vi "REV Sequence.vi"() -> ()   [LabVIEW 2026]
uses:
  <vilib>/REVLibDriver5/subvi/RevLibError.ctl
  <vilib>/Custom Controls/c_Spark_MotorType.ctl
  <vilib>/REVLibDriver5/REVLibDriver.lvlib
  <vilib>/Custom Controls/c_Spark_SparkModel.ctl
  lib/libREVLibDriver.so
panel:
  out "c_Spark_SparkModel":T1 items=["c_Spark_Unknown", "c_Spark_SparkFlex", "c_Spark_SparkMax"]
  out "function return 4":T2
  out "fwVersion out":T3
  in  "stop":bool
  out "function return 3":T2
  out "function return 2":T2
  out "function return":T2
  out "deviceId out":i32
  out "status out":T2
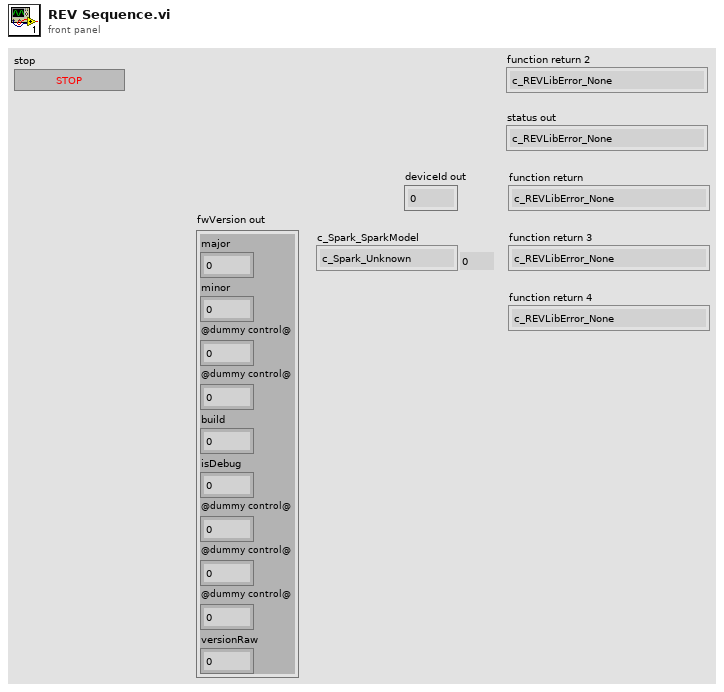
[diagram p1: front panel]
types:
  T1 = typedef "REVLibDriver.lvlib/c_Spark_SparkModel.ctl" = u16
  T2 = typedef "REVLibDriver.lvlib/RevLibError.ctl" = enum16{"c_REVLibError_None", "c_REVLibError_General", "c_REVLibError_CANTimeout", "c_REVLibError_NotImplemented", "c_REVLibError_HAL", "c_REVLibError_CantFindFirmware", "c_REVLibError_FirmwareTooOld", "c_REVLibError_FirmwareTooNew", "c_REVLibError_ParamInvalidID", "c_REVLibError_ParamMismatchType", "c_REVLibError_ParamAccessMode", "c_REVLibError_ParamInvalid", "c_REVLibError_ParamNotImplementedDeprecated", "c_REVLibError_FollowConfigMismatch", "c_REVLibError_Invalid", "c_REVLibError_SetpointOutOfRange", "c_REVLibError_Unknown", "c_REVLibError_CANDisconnected", "c_REVLibError_DuplicateCANId", "c_REVLibError_InvalidCANId", "c_REVLibError_SparkMaxDataPortAlreadyConfiguredDifferently", "c_REVLibError_SparkFlexBrushedWithoutDock", "c_REVLibError_InvalidBrushlessEncoderConfiguration", "c_REVLibError_FeedbackSensorIncompatibleWithDataPortConfig", "c_REVLibError_ParamInvalidChannel", "c_REVLibError_ParamInvalidValue", "c_REVLibError_CannotPersistParametersWhileEnabled", "c_REVLibError_NotReadyToReceiveCommand", "c_REVLibError_NumCodes"}
  T3 = cluster{"major":u8, "minor":u8, "@dummy control@":i8, "@dummy control@":i8, "build":u32, "isDebug":u8, "@dummy control@":i8, "@dummy control@":i8, "@dummy control@":i8, "versionRaw":u32}
  T4 = typedef "REVLibDriver.lvlib/c_Spark_MotorType.ctl" = enum16{"c_Spark_kMotorType_BRUSHED", "    c_Spark_kMotorType_BRUSHLESS", "    c_Spark_kNumMotorTypes"}
  T5 = typedef "REVLibDriver.lvlib/c_Spark_handle.ctl" = cluster{"Pointer":u64}
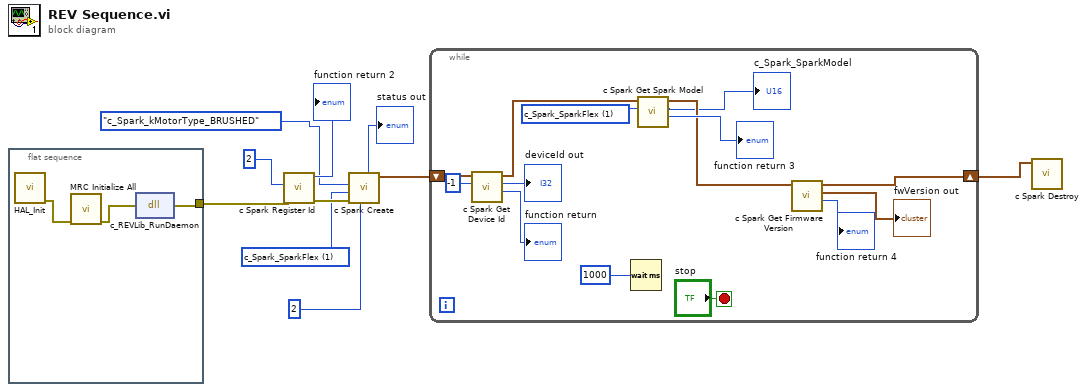
[diagram p0: block diagram]
diagram:
  w9 = T1 1 items=["c_Spark_SparkMax"=0, "c_Spark_SparkFlex"=1, "c_Spark_Unknown"=255] ("unconfirmedModel")
  n1 = flat-sequence {
    tunnel: [w13] -> w3
    frame #0 {
      n2 = call "HAL_Init.vi"() -> ("error out"=w12:errorcluster)  [unwired: 11 in]
      n3 = call <vilib>:"MRC Initialize All.vi"("error out 2"=w12) -> ("error out"=w11:errorcluster)  [unwired: 10 in]
      n4 = dll-call lib="home/systemcore/natinst/lib/libREVLibDriver.so" fn="c_REVLib_RunDaemon"(error in=w11) -> (error out=w13:errorcluster)  [unwired: 3 in, 1 out]
    }
  }
  n5 = call <vilib>:"c Spark Register Id.vi"("error in (no error)"=w3, "deviceId"=2) -> ("error out"=w10:errorcluster, "function return"=→"function return 2":T2)  [unwired: 8 in]
  n6 = call <vilib>:"c Spark Create.vi"("deviceId"=2, "error in (no error)"=w10, "unconfirmedModel"=w9, "type"=c_Spark_MotorType."c_Spark_kMotorType_BRUSHED") -> ("handle"=w6:T5, "status out"=→"status out":T2)  [unwired: 5 in, 1 out]
  n7 = while {
    shift-right: [w15] -> w2
    shift-left: w6 -> [w27]
    stop <- "stop" stop-if-true
    w16 = T1 1 items=["c_Spark_Unknown", "c_Spark_SparkFlex", "c_Spark_SparkMax"] ("model")
    n8 = call <vilib>:"c Spark Get Device Id.vi"("deviceId"=-1, "handle"=w27) -> ("function return"=→"function return":T2, "deviceId out"=→"deviceId out":i32, "handle out"=w24:T5)  [unwired: 6 in, 1 out]
    n9 = Wait (ms)(milliseconds to wait=u32 1000) -> ()  [unwired: 1 out]
    n10 = call <vilib>:"c Spark Get Spark Model.vi"("c_Spark_SparkModel"=w16, "handle"=w24) -> ("function return"=→"function return 3":T2, "c_Spark_SparkModel"=→"c_Spark_SparkModel":T1, "handle out"=w20:T5)  [unwired: 6 in, 1 out]
    n11 = call <vilib>:"c Spark Get Firmware Version.vi"("handle"=w20) -> ("function return"=→"function return 4":T2, "fwVersion out"=→"fwVersion out":T3, "handle out"=w15:T5)  [unwired: 7 in, 1 out]
  }
  n12 = call <vilib>:"c Spark Destroy.vi"("handle"=w2) -> ()  [unwired: 9 in, 2 out]
